vi "testParseStateQueueError.vi"(8 "error in (no error)":errorcluster, 11 "testStateMachineUtilities in":refnum<class "testStateMachineUtilities.lvclass">=refnum) -> (0 "error out":errorcluster, 3 "testStateMachineUtilities out":refnum<class "testStateMachineUtilities.lvclass">)   [LabVIEW 2016, in "testStateMachineUtilities.lvclass"]
uses:
  testStateMachineUtilities.lvclass
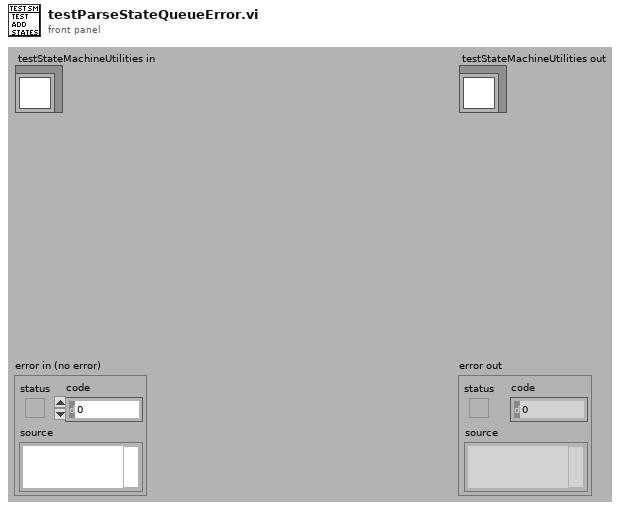
[diagram p1: front panel]
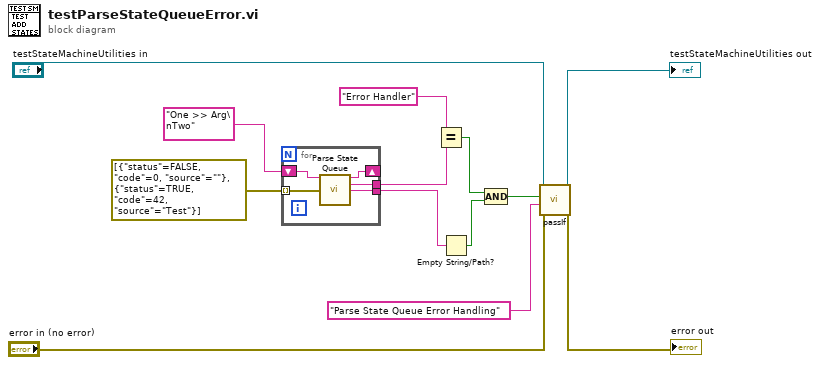
[diagram p0: block diagram]
diagram:
  n1 = for {
    tunnel: errorcluster[] [{"status"=FALSE, "code"=0, "source"=""}, {"status"=TRUE, "code"=42, "source"="Test"}] -> [w18] mode=indexing
    tunnel: [w16] -> w6
    tunnel: [w15] -> w7
    shift-right: [w14] -> _
    shift-left: "One >> Arg\nTwo" ("State Queue") -> [w17]
    n2 = call "Parse State Queue.vi"("State Queue"=w17, "Error In (no error)"=w18) -> ("Remaining States"=w14:string, "Current State"=w15:string, "Arguments"=w16:string)  [unwired: 11 in]
  }
  n3 = Equal?(x="Error Handler", y=w7) -> (x = y?=w5:bool)
  n4 = Empty String/Path?(string/path=w6) -> (empty?=w2:bool)
  n5 = Compound Arithmetic op=AND(w5, w2) -> (w4:bool)
  n6 = call-dynamic "passIf.vi"("error in (no error)"="error in (no error)", "message (\"\")"="Parse State Queue Error Handling", "pass"=w4, "TestCase in"="testStateMachineUtilities in") -> ("error out"=→"error out":errorcluster, "TestCase out"=→"testStateMachineUtilities out":refnum<class "testStateMachineUtilities.lvclass">)  [unwired: 6 in]
